vi "Untitled 4.vi"() -> ()   [LabVIEW 2023]
uses:
  Timer_Operation_Select.ctl
panel:
  out "Error_Out":errorcluster
  out "T4_Time_Out? 4":bool
  out "T3_Time_Out? 3":bool
  out "T2_Time_Out? 2":bool
  out "T1_Time_Out?":bool
  in  "Timer_Select":T1=enum."Start_Timer"
  in  "Error_In":errorcluster
  in  "T4_Start?":bool
  in  "T3_Start?":bool
  in  "T2_Start?":bool
  in  "Wait_Time":dbl=10.0 format="%#_13g"
  in  "T1_Start?":bool
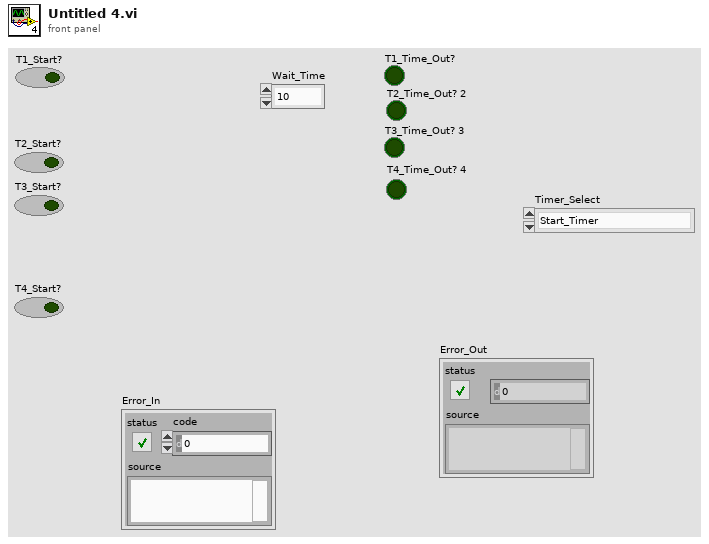
[diagram p1: front panel]
types:
  T1 = typedef "Timer_Operation_Select.ctl" = enum16{"Initialize", "Start_Timer", "Time_Out?", "Stop_Timer"}
  T2 = typedef "Timer_Data_Out.ctl" = cluster{"T1_Time":dbl, "T1_Time_Out?":bool, "T2_Time":dbl, "T2_Time_Out?":bool, "T3_Time":dbl, "T3_Time_Out":bool, "T4_Time":dbl, "T4_Time_Out":bool}
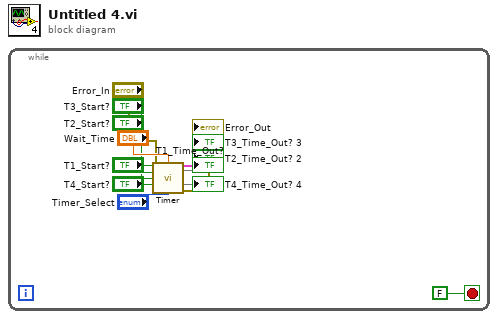
[diagram p0: block diagram]
diagram:
  n1 = while {
    stop <- FALSE stop-if-true
    n2 = call "Timer.vi"("Timers_Start"="T1_Start?", "Wait_Time"="Wait_Time", 5:"T2_Start?", 7:"T3_Start?", 9:"T4_Start?", "Error_In"="Error_In", "Timer_Select"="Timer_Select") -> ("Timer_Data_Out"=→"T1_Time_Out?":T2, 6:→"T2_Time_Out? 2", 8:→"T3_Time_Out? 3", 10:→"T4_Time_Out? 4", "Error_Out"=→"Error_Out":errorcluster)  [unwired: 4 in]
  }
